vi "Configure Parent Class.vi"(8 "error in (no error)":errorcluster, 10 "Parent Class":string, 11 "New Class Dialog In":refnum<class "New Class Dialog.lvclass">) -> (0 "error out":errorcluster, 3 "New Class Dialog Out":refnum<class "New Class Dialog.lvclass">)   [LabVIEW 2020, in "Process Generation.lvlib" / "New Class Dialog.lvclass"]
uses:
  New Class Dialog.lvclass
  Framework/Process/Process.lvclass
  New Class Dialog.lvclass/New Class Dialog.ctl
  Process Generator/Process Generator.lvclass/Process Generator.ctl
  Process Generator/Process Generator.lvclass
  Framework Test/Process Test/Process Test.lvclass
  C:/Users/anton/Documents/GitHub/Triarc-Framework/source/Framework Test/Base Class Test/Base Test.lvclass
  C:/Program Files (x86)/National Instruments/LabVIEW 2020/vi.lib/Asteme/LUnit/Test Case.lvclass
  C:/Users/anton/Documents/GitHub/Triarc-Framework/source/Framework Test/Process Test/Process Test.lvclass
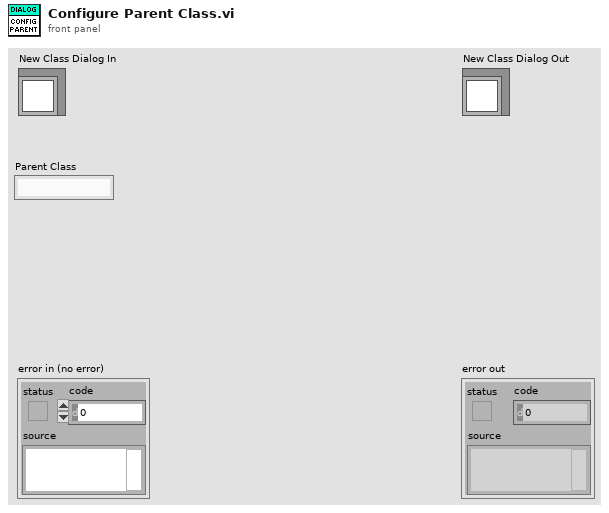
[diagram p1: front panel]
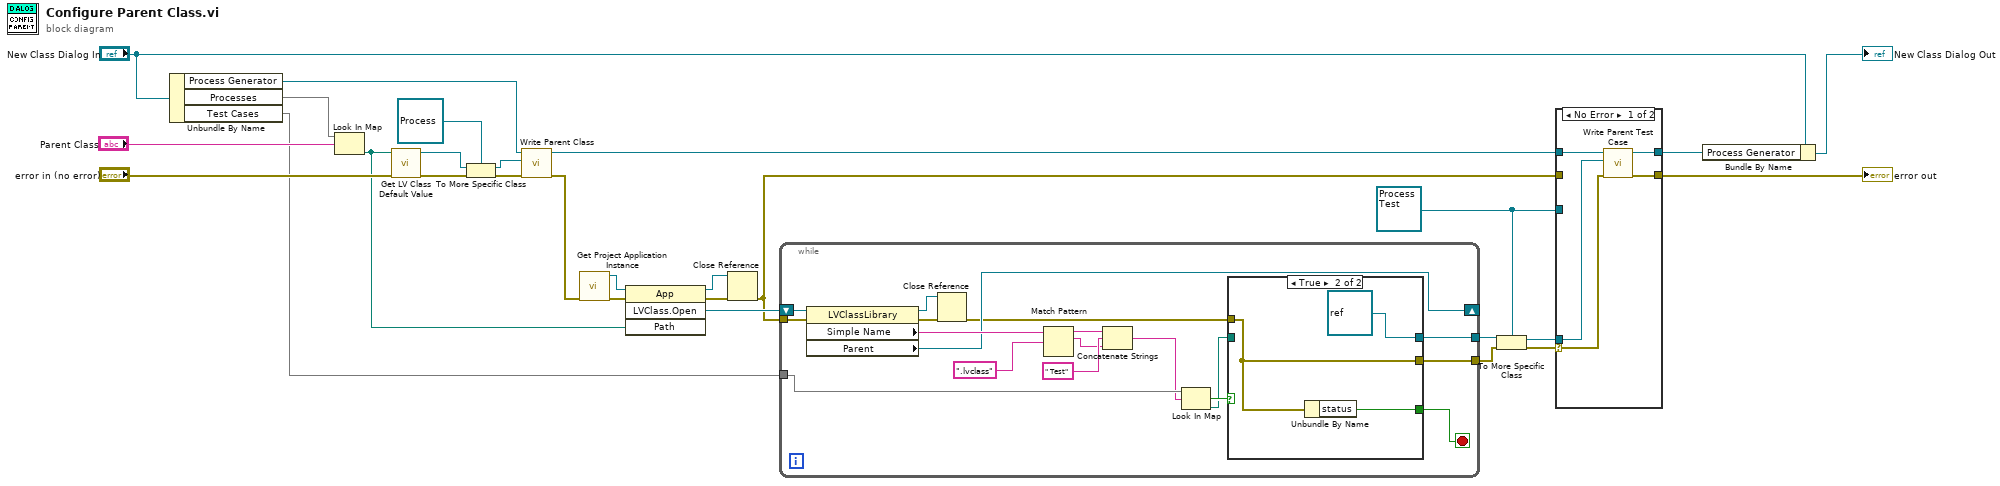
[diagram p0: block diagram]
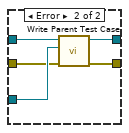
[diagram p2: hidden frame]
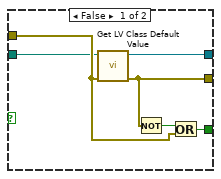
[diagram p3: hidden frame]
diagram:
  w5 = refnum<class "Process Test.lvclass"> refnum ("Process Test.lvclass")
  n1 = Unbundle By Name("New Class Dialog In") -> ("Process Generator"=w20:refnum<class "Process Generator.lvclass">, "Processes"=w28:map{string, path}, "Test Cases"=w3:map{string, path})
  n2 = Look In Map(map=w28, key="Parent Class") -> (value=w17:path)  [unwired: 1 in, 1 out]
  n3 = call <vilib>:"Get LV Class Default Value.vi"("error in (no error)"="error in (no error)", "class path"=w17) -> ("error out"=w22:errorcluster, "object"=w24:refnum<class>)  [unwired: 8 in]
  n4 = To More Specific Class(target class=refnum<class "Process.lvclass"> refnum ("Parent Process"), reference=w24, error in=w22) -> (specific class reference=w26:refnum<class "Process.lvclass">, error out=w21:errorcluster)
  n5 = call "Write Parent Class.vi"("error in (no error)"=w21, "Parent Process"=w26, "Process Generator in"=w20) -> ("error out"=w13:errorcluster, "Process Generator out"=w11:refnum<class "Process Generator.lvclass">)  [unwired: 7 in]
  n6 = call "Get Project Application Instance.vi"("error in (no error)"=w13) -> ("error out"=w15:errorcluster, "Application out"=w16:refnum<vi>)  [unwired: 9 in]
  n7 = invoke class="App" method="LVClass.Open"(reference=w16, error in=w15, "Path"=w17) -> (reference out=w2:refnum<vi>, error out=w1:errorcluster, "LVClass.Open"=w14:refnum<vi>)  [unwired: 1 in, 1 out]
  n8 = Close Reference(reference=w2, error in (no error)=w1) -> (error out=w4:errorcluster)
  n9 = while {
    tunnel: w4 -> [w45]
    tunnel: [w37] -> w12
    shift-right: [w36] -> _
    shift-left: w14 -> [w46]
    tunnel: [w33] -> w7
    tunnel: w3 -> [w32]
    stop <- w35 stop-if-true
    n10 = property class="LVClassLibrary"(reference=w46, error in=w45) -> (reference out=w38:refnum<vi>, error out=w39:errorcluster, "Simple Name"=w44:string, "Parent"=w36:refnum<vi>)
    n11 = Close Reference(reference=w38, error in (no error)=w39) -> (error out=w34:errorcluster)
    n12 = Match Pattern(string=w44, regular expression=".lvclass") -> (before substring=w42:string, match substring=w40:string)  [unwired: 1 in, 2 out]
    n13 = Concatenate Strings(w42, " Test" ("string"), w40) -> (w31:string)
    n14 = Look In Map(map=w32, key=w31) -> (key not found?=w30:bool, value=w29:path)  [unwired: 1 in]
    n15 = case shown="True" w30 {
      tunnel: [w52 refnum<class> refnum ("object")] -> w37
      tunnel: [w51 w53] -> w35
      tunnel: w34 -> [w49 w54]
      tunnel: [w48 w54] -> w33
      tunnel: w29 -> [w47 _]
      frame False {
        n16 = call <vilib>:"Get LV Class Default Value.vi"("error in (no error)"=w49, "class path"=w47) -> ("error out"=w48:errorcluster, "object"=w52:refnum<class>)  [unwired: 8 in]
        n17 = Not(x=w48) -> (.not. x?=w50:bool)
        n18 = Or(x=w50, y=w49) -> (x .or. y?=w51:bool)
      }
      frame True {
        n19 = Unbundle By Name(w54) -> ("status"=w53:bool)
      }
    }
  }
  n20 = To More Specific Class(target class=w5, reference=w12, error in=w7) -> (specific class reference=w9:refnum<class "Process Test.lvclass">, error out=w8:errorcluster)
  n21 = case shown="No Error" w8 {
    selector: w8 -> [w57 _]
    tunnel: w11 -> [w60 w65]
    tunnel: [w59 w64] -> w10
    tunnel: w9 -> [w58 _]
    tunnel: [w56 w63] -> w6
    tunnel: w5 -> [_ w62]
    tunnel: w4 -> [_ w61]
    frame No Error {
      n22 = call "Write Parent Test Case.vi"("error in (no error)"=w57, "Parent Test Case"=w58, "Process Generator In"=w60) -> ("error out"=w56:errorcluster, "Process Generator Out"=w59:refnum<class "Process Generator.lvclass">)  [unwired: 7 in]
    }
    frame Error {
      n23 = call "Write Parent Test Case.vi"("error in (no error)"=w61, "Parent Test Case"=w62, "Process Generator In"=w65) -> ("error out"=w63:errorcluster, "Process Generator Out"=w64:refnum<class "Process Generator.lvclass">)  [unwired: 7 in]
    }
  }
  "error out" <- w6
  n24 = Bundle By Name(cluster="New Class Dialog In", "Process Generator"=w10) -> (→"New Class Dialog Out":refnum<class "New Class Dialog.lvclass">)
